vi "ComboBox-Update Strings.vi"(0 "ComboBox in":refnum<vi>, 7 "NewVal":string, 11 "error in (no error)":errorcluster) -> (4 "reference out":refnum<vi>, 6 "Strings[]":string[](array[string]), 10 "new?":bool, 15 "error out":errorcluster)   [LabVIEW 2020]
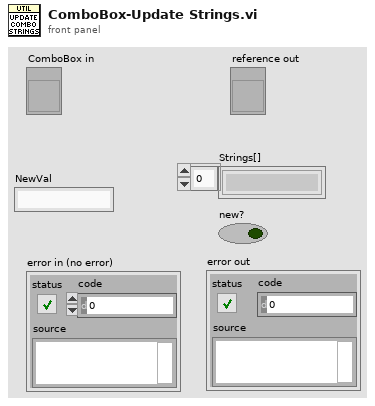
[diagram p1: front panel]
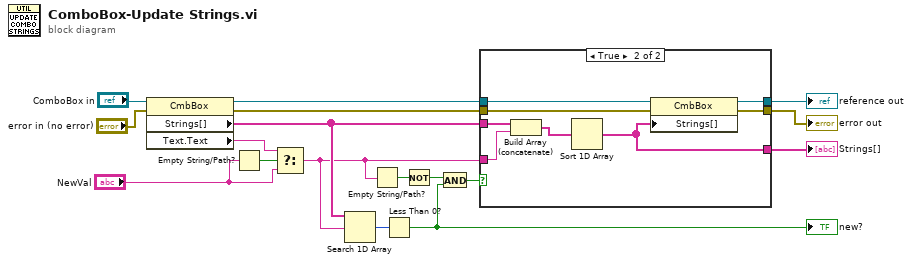
[diagram p0: block diagram]
diagram:
  n1 = property class="CmbBox"(reference="ComboBox in", error in="error in (no error)") -> (reference out=w14:refnum<vi>, error out=w13:errorcluster, "Strings[]"=w2:string[], "Text.Text"=w8:string)
  n2 = Empty String/Path?(string/path="NewVal") -> (empty?=w9:bool)
  n3 = Select(t=w8, s=w9, f="NewVal") -> (s? t:f=w1:string)
  n4 = Search 1D Array(1D array=w2, element=w1) -> (index of element=w15:i32)  [unwired: 1 in]
  n5 = Empty String/Path?(string/path=w1) -> (empty?=w4:bool)
  n6 = Less Than 0?(x=w15) -> (x < 0?=w6:bool)
  "new?" <- w6
  n7 = Not(x=w4) -> (.not. x?=w3:bool)
  n8 = And(x=w3, y=w6) -> (x .and. y?=w5:bool)
  n9 = case shown="True" w5 {
    tunnel: w14 -> [w19 w27]
    tunnel: w13 -> [w18 w26]
    tunnel: w2 -> [w20 w28]
    tunnel: [w19 w25] -> w12
    tunnel: [w18 w24] -> w11
    tunnel: [w20 w21] -> w10
    tunnel: w1 -> [_ w23]
    frame False {
    }
    frame True {
      n10 = Build Array (concatenate)(w28, w23) -> (w22:string[])
      n11 = Sort 1D Array(array=w22) -> (sorted array=w21:string[])
      n12 = property class="CmbBox"(reference=w27, error in=w26, "Strings[]"=w21) -> (reference out=w25:refnum<vi>, error out=w24:errorcluster)
    }
  }
  "Strings[]" <- w10
  "reference out" <- w12
  "error out" <- w11
